vi "Read Scope Setting.vi"(8 "error in (no error)":errorcluster, 11 "Scope configuration":refnum<class "Scope configuration.lvclass">) -> (0 "error out":errorcluster, 2 "Scope Setting":T1={"Sampling Rate"=10000000.0, "Number of Samples"=1000000, "Type"="Window - Entering", "Pretrigger"=10.0, "Source"="CH0", "Level 1"=1.0, "Level 2"=10.0, "Trigger Coupling"="DC", "TrigDest"="None", "Group"="None"} {"Level 2" format="%#_6p"; "Level 1" format="%#_6p"; "Pretrigger" format="%#_f"; "Number of Samples" format="%#_6p"; "Sampling Rate" format="%#_6p"}, 3 "Scope configuration out":refnum<class "Scope configuration.lvclass">)   [LabVIEW 2025, in "Scope.lvlib" / "Scope configuration.lvclass"]
uses:
  Scope configuration.lvclass
  Scope Instrument Setting.ctl
  Scope configuration.lvclass/Scope configuration.ctl
panel:
  # "Trigger"
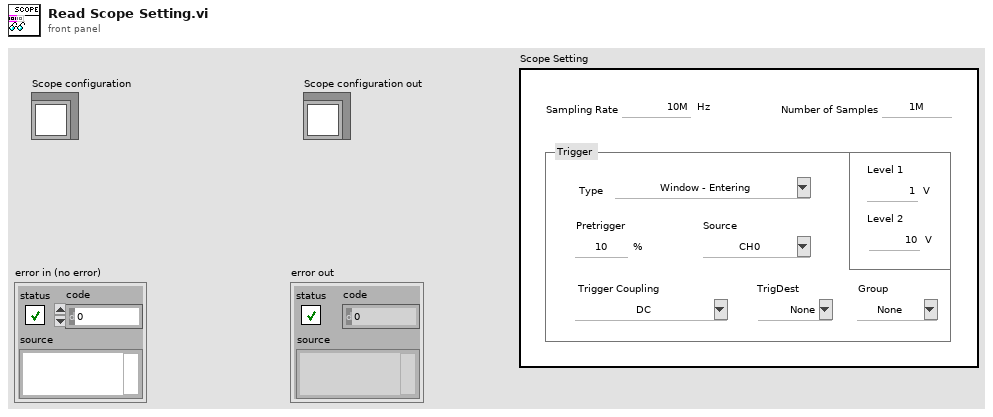
[diagram p1: front panel]
types:
  T1 = typedef "Scope.lvlib/Scope configuration.lvclass/Scope Instrument Setting.ctl" = cluster{"Sampling Rate":dbl, "Number of Samples":u32, "Type":string, "Pretrigger":dbl, "Source":string, "Level 1":dbl, "Level 2":dbl, "Trigger Coupling":string, "TrigDest":string, "Group":string}
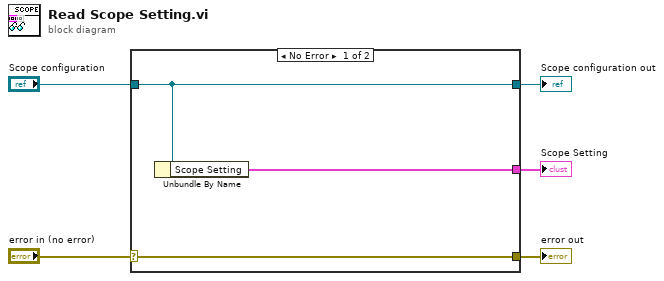
[diagram p0: block diagram]
diagram:
  n1 = case shown="No Error" "error in (no error)" {
    selector: "error in (no error)" -> [w8 w9]
    tunnel: [w8 w9] -> w4
    tunnel: [w7 w10] -> w2
    tunnel: "Scope configuration" -> [w7 w10]
    tunnel: [w6 _] -> w1
    frame No Error {
      n2 = Unbundle By Name(w7) -> ("Scope Setting"=w6:T1)
    }
    frame Error {
    }
  }
  "error out" <- w4
  "Scope configuration out" <- w2
  "Scope Setting" <- w1
